vi "BoolCmd_Multiplexor.vi"(6 "Ready":bool=TRUE, 8 "Command Cancel":bool, 9 "Command 3":bool, 10 "Command 2":bool, 11 "Command 1":bool) -> (0 "Do Command 3":bool, 1 "Do Cancel 2":bool, 2 "Do Command 2":bool, 3 "Do Cancel 1":bool, 4 "Do Cancel 3":bool, 5 "Do Command 1":bool)   [LabVIEW 2019, in "Trajectory_Library.lvlib"]
uses:
  Trajectory_Library.lvlib
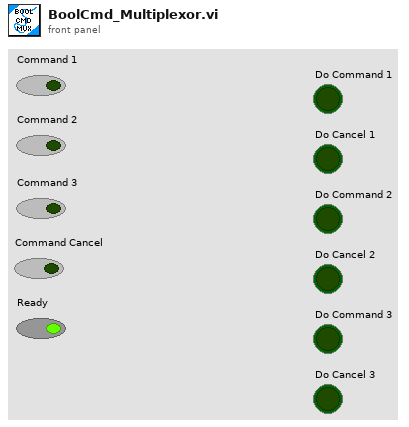
[diagram p1: front panel]
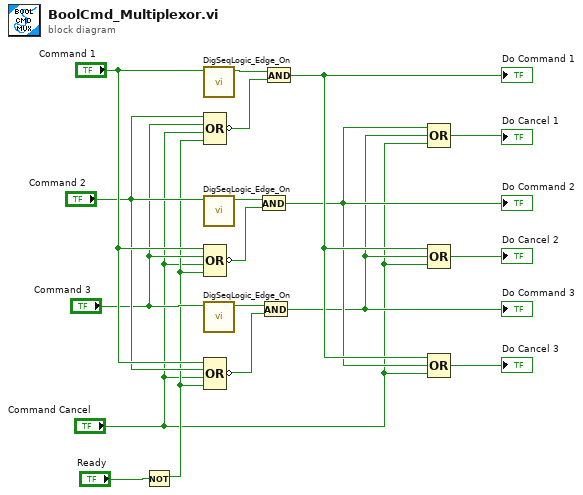
[diagram p0: block diagram]
diagram:
  n1 = Not(x="Ready") -> (.not. x?=w12:bool)
  n2 = call "DigSeqLogic_Edge_On.vi"("Input"="Command 1") -> ("On Edge"=w15:bool)  [unwired: 10 in]
  n3 = Compound Arithmetic op=OR("Command 2", "Command 3", "Command Cancel", w12) -> (invert w14:bool)
  n4 = call "DigSeqLogic_Edge_On.vi"("Input"="Command 2") -> ("On Edge"=w11:bool)  [unwired: 10 in]
  n5 = Compound Arithmetic op=OR("Command 1", "Command 3", "Command Cancel", w12) -> (invert w10:bool)
  n6 = call "DigSeqLogic_Edge_On.vi"("Input"="Command 3") -> ("On Edge"=w9:bool)  [unwired: 10 in]
  n7 = Compound Arithmetic op=OR("Command 1", "Command 2", "Command Cancel", w12) -> (invert w8:bool)
  n8 = And(x=w11, y=w10) -> (x .and. y?=w4:bool)
  "Do Command 2" <- w4
  n9 = And(x=w9, y=w8) -> (x .and. y?=w2:bool)
  "Do Command 3" <- w2
  n10 = And(x=w15, y=w14) -> (x .and. y?=w7:bool)
  "Do Command 1" <- w7
  n11 = Compound Arithmetic op=OR(w4, w2, "Command Cancel") -> (→"Do Cancel 1":bool)
  n12 = Compound Arithmetic op=OR(w7, w2, "Command Cancel") -> (→"Do Cancel 2":bool)
  n13 = Compound Arithmetic op=OR(w7, w4, "Command Cancel") -> (→"Do Cancel 3":bool)
